vi "Write.vi"() -> ()   [LabVIEW 2013]
uses:
  <vilib>/NI/Modbus Library/API/Master/Modbus Master.lvclass
  <vilib>/NI/Modbus Library/API/Wrapper/Create TCP Master.vi
  GlobalStop.vi
  <vilib>/NI/Modbus Library/API/Wrapper/API Main.lvlib
panel:
  out "error out":errorcluster
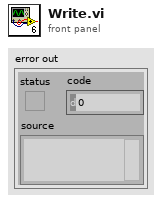
[diagram p1: front panel]
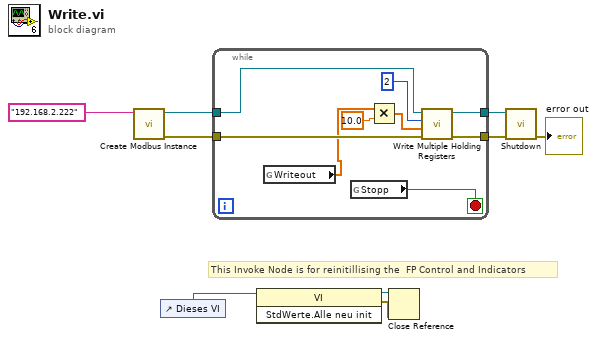
[diagram p0: block diagram]
diagram:
  # "This Invoke Node is for reinitillising the  FP Control and Indicators"
  n1 = call-poly <vilib>:"Create Modbus Instance.vi"("address"="192.168.2.222") -> ("error out"=w9:errorcluster, "TCP master instance"=w6:refnum<class "Modbus Master.lvclass">)  [unwired: 9 in]
  n2 = control-ref of="Dieses VI"() -> (w3:refnum<vi>)
  n3 = while {
    tunnel: w9 -> [w18]
    tunnel: [w17] -> w8
    tunnel: [w16] -> w7
    tunnel: w6 -> [w15]
    stop <- w10 stop-if-true
    n4 = global read "GlobalWrite.vi" "Writeout"() -> (w11:dbl[])
    n5 = global read "GlobalStop.vi" "Stopp"() -> (w10:bool)
    n6 = Multiply(x=w11, y=10.0) -> (x*y=w12:dbl[])
    n7 = call-dynamic "Write Multiple Holding Registers.vi"("error in"=w18, "registers to write"=w12, "starting address"=u16 2, "Modbus master in"=w15) -> ("error out"=w17:errorcluster, "Modbus master out"=w16:refnum<class "Modbus Master.lvclass">)  [unwired: 6 in]
  }
  n8 = invoke class="VI" method="StdWerte.Alle neu init"(reference=w3) -> (reference out=w2:refnum<vi>, error out=w1:errorcluster)  [unwired: 2 in, 1 out]
  n9 = Close Reference(reference=w2, error in (no error)=w1) -> ()  [unwired: 1 out]
  n10 = call-dynamic "Shutdown.vi"("error in"=w8, "Modbus master in"=w7) -> ("error out"=→"error out":errorcluster)  [unwired: 9 in]
